vi "GetValue.vi"(8 "error in":errorcluster, 11 "ExecutionStatus in":refnum<class "ExecutionStatus.lvclass">) -> (0 "error out":errorcluster, 2 "Value":T1=enum."NOT_COMPLETED", 3 "ExecutionStatus out":refnum<class "ExecutionStatus.lvclass">)   [LabVIEW 2021, in "ProligentXMLGenerator.lvlib" / "ExecutionStatus.lvclass"]
uses:
  ExecutionStatus.lvclass
  ExecutionStatus.lvclass/ExecutionStatus.ctl
  Value.ctl
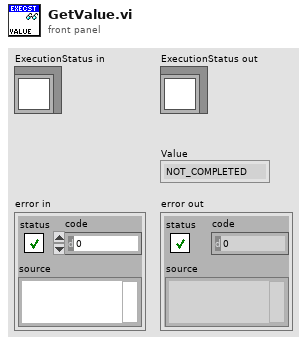
[diagram p1: front panel]
types:
  T1 = typedef "ProligentXMLGenerator.lvlib/ExecutionStatus.lvclass/Value.ctl" = enum16{"PASS", "FAIL", "NOT_COMPLETED", "ABORTED"}
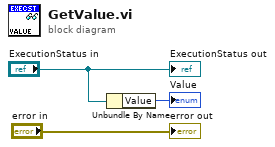
[diagram p0: block diagram]
diagram:
  n1 = Unbundle By Name("ExecutionStatus in") -> ("Value"=→"Value":T1)
  "error out" <- "error in"
  "ExecutionStatus out" <- "ExecutionStatus in"
